vi "InstrumentsOn.vi"() -> ()   [LabVIEW 2019]
panel:
  in  "Attocubes On?":bool
  in  "PZC200 On?":bool
  in  "Cryostation On?":bool
  in  "PM16-120 On?":bool
  in  "PicoHarp On?":bool
  in  "LightField On?":bool
  in  "ESP 300 On?":bool
  in  "KCubes Piezo On?":bool
  in  "KCube Shutter On?":bool
  in  "ESP 301 On?":bool
  in  "FSM 300 On?":bool
  in  "Laser Comm On?":bool
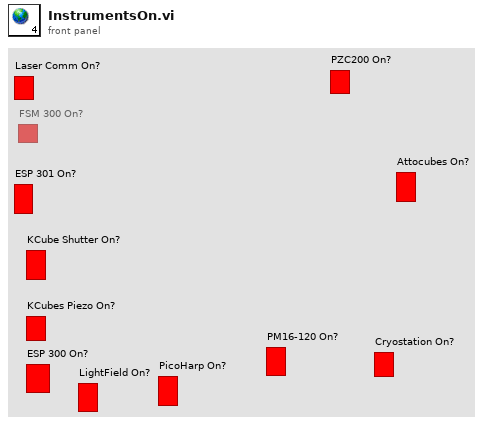
[diagram p1: front panel]
diagram:
